vi "Send Set Reference Range COM Port.vi"(7 "Priority":T1=enum."Normal" caption="Message Priority (Normal)", 8 "error in (no error)":errorcluster, 10 "Reference Range COM Port":refnum<visa-resource-name>, 11 "Message Enqueuer in":refnum<class "Message Enqueuer.lvclass">) -> (0 "error out":errorcluster, 3 "Message Enqueuer out":refnum<class "Message Enqueuer.lvclass">)   [LabVIEW 2017, in "Set Reference Range COM Port Msg.lvclass"]
doc: "Sends the <b>Reference Range.lvlib:Set Reference Range COM Port Msg.lvclass</b> message.\n\nThis message will call <b>Set Reference Range COM Port.vi</b> on the <b>Reference Range.lvlib:Reference Range Actor.lvclass</b> actor.\n\n<b>Set Reference Range COM Port.vi Description</b>"
uses:
  Set Reference Range COM Port Msg.lvclass
  <vilib>/ActorFramework/Message Enqueuer/Message Enqueuer.lvclass
  <vilib>/ActorFramework/Message Enqueuer/Message Priority.ctl
  C:/Program Files (x86)/National Instruments/LabVIEW 2017/vi.lib/ActorFramework/Message/Message.lvclass
  Set Reference Range COM Port Msg.lvclass/Set Reference Range COM Port Msg.ctl
  <vilib>/ActorFramework/Message Enqueuer/Message Enqueuer.lvclass/Message Enqueuer.ctl
  <vilib>/ActorFramework/Message Priority Queue/Priority Enqueue.vi
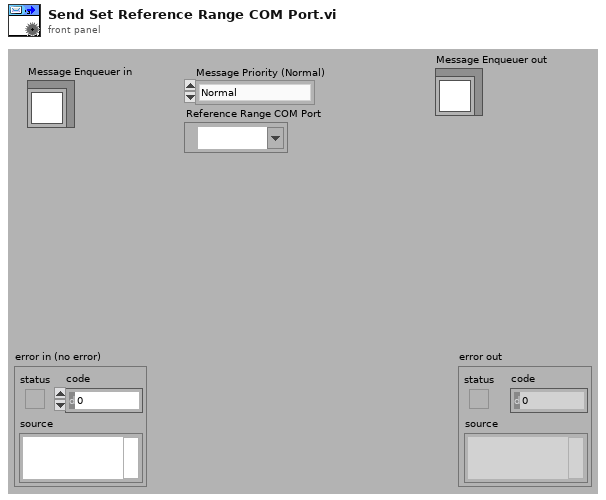
[diagram p1: front panel]
types:
  T1 = typedef "Actor Framework.lvlib/Message Enqueuer.lvclass/Message Priority.ctl" = enum16{"Low", "Normal", "High"}
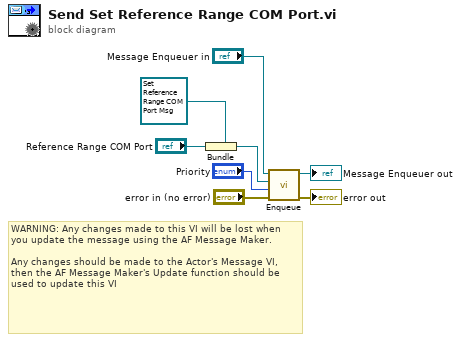
[diagram p0: block diagram]
diagram:
  # "WARNING: Any changes made to this VI will be lost when you update the message using the AF Message Maker.\n\nAny changes should be made to the Actor's Message VI, then the AF Message Maker's Update function should be used to update this VI"
  n1 = Bundle(cluster=refnum<class "Set Reference Range COM Port Msg.lvclass"> refnum ("Reference Range.lvlib:Set Reference Range COM Port Msg.lvclass"), "Reference Range COM Port") -> (w4:refnum<class "Set Reference Range COM Port Msg.lvclass">)
  n2 = call <vilib>:"Enqueue.vi"("error in (no error)"="error in (no error)", "Message Priority (Normal)"="Priority", "Message"=w4, "Message Enqueuer in"="Message Enqueuer in") -> ("error out"=→"error out":errorcluster, "Message Enqueuer out"=→"Message Enqueuer out":refnum<class "Message Enqueuer.lvclass">)  [unwired: 6 in]
